vi "Get Multiple Entries.vi"(8 "error in (no error)":errorcluster, 10 "Keys":string[](array[string]) caption="Names", 11 "Registry in":refnum<class "Registry.lvclass">) -> (0 "error out":errorcluster, 1 "Values":variant[](array[variant]), 2 "Keys":string[](array[string]) caption="Names", 4 "Found?":bool[](array[boolean]))   [LabVIEW 2020, in "BCI-1553 API.lvlib" / "Registry.lvlib" / "Registry.lvclass"]
doc: "Retrieves multiple Key/Value pairs from the Registry."
uses:
  Registry.lvclass
  Registry.lvclass/Registry.ctl
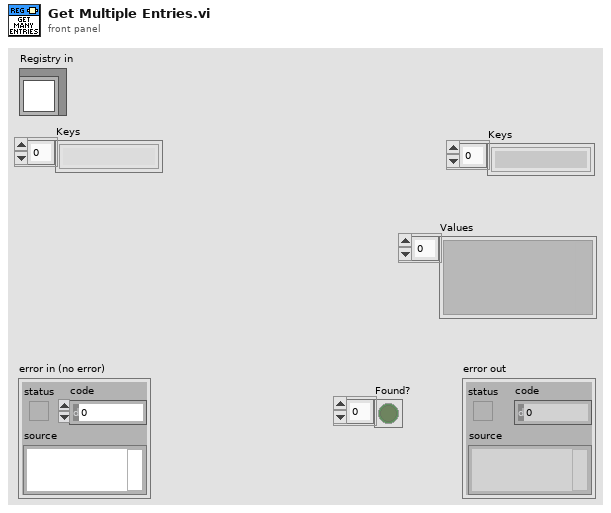
[diagram p1: front panel]
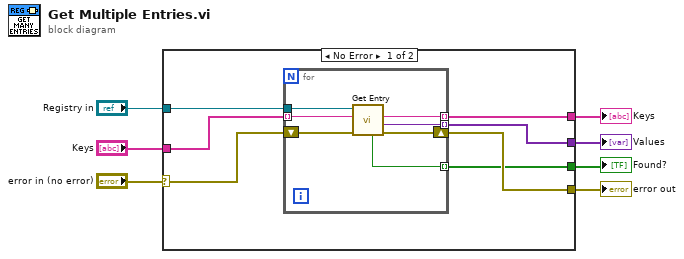
[diagram p0: block diagram]
diagram:
  n1 = case shown="No Error" "error in (no error)" {
    selector: "error in (no error)" -> [w14 w22]
    tunnel: [w13 w22] -> w6
    tunnel: "Registry in" -> [w8 _]
    tunnel: "Keys" -> [w12 _]
    tunnel: [w11 _] -> w3
    tunnel: [w10 _] -> w2
    tunnel: [w9 _] -> w1
    frame No Error {
      n2 = for {
        shift-right: [w20] -> w13
        shift-left: w14 -> [w21]
        tunnel: w12 -> [w19] mode=indexing
        tunnel: [w18] -> w11 mode=indexing
        tunnel: [w17] -> w10 mode=indexing
        tunnel: [w16] -> w9 mode=indexing
        tunnel: w8 -> [w15]
        n3 = call "Get Entry.vi"("error in (no error)"=w21, "Key"=w19, "Registry in"=w15) -> ("error out"=w20:errorcluster, "Value"=w17:variant, "Key Out"=w18:string, "Found?"=w16:bool)  [unwired: 5 in]
      }
    }
    frame Error {
    }
  }
  "error out" <- w6
  "Keys" <- w3
  "Values" <- w2
  "Found?" <- w1
